vi "Helper - ManualSails.vi"(0 "Full In":bool, 1 "Sheet In":bool, 2 "Sheet Out":bool, 3 "Full Out":bool, 4 "Array":dbl[](array[numeric])) -> (5 "Array 2":dbl[](array[numeric]))   [LabVIEW 2011]
panel:
  # "This is the output array, but it\nnever gets veiwed"
  # "This control gets passed\nan array"
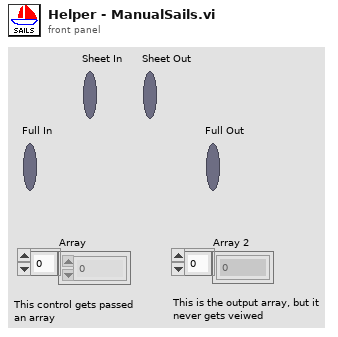
[diagram p1: front panel]
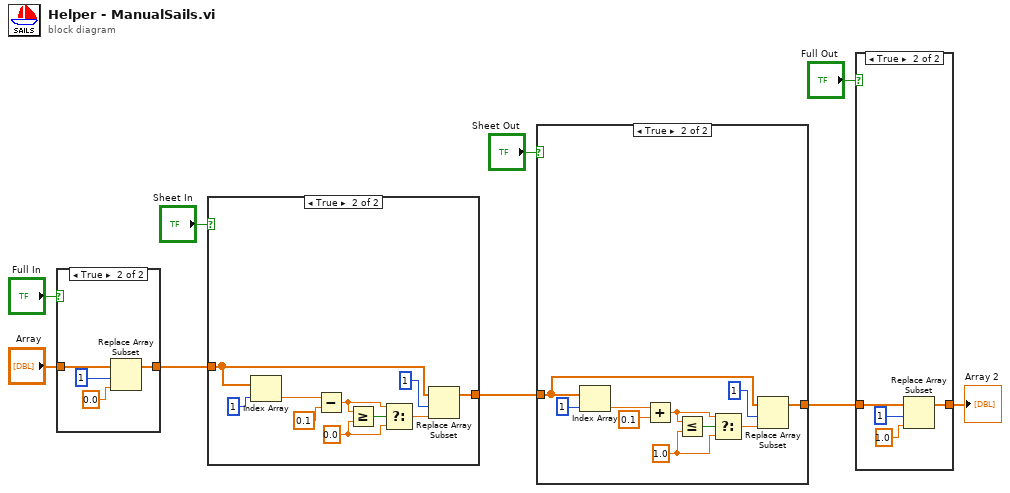
[diagram p0: block diagram]
diagram:
  n1 = case shown="True" "Full In" {
    tunnel: "Array" -> [w10 w14]
    tunnel: [w10 w12] -> w8
    frame False {
    }
    frame True {
      n2 = Replace Array Subset(array=w14, new element=0.0 ("new element/subarray"), index=1) -> (w12:dbl[])
    }
  }
  n3 = case shown="True" "Sheet In" {
    tunnel: w8 -> [w15 w24]
    tunnel: [w15 w25] -> w7
    frame False {
    }
    frame True {
      w20 = 0.0 ("y")
      n4 = Index Array(array=w24, index=1) -> (element=w17:dbl)
      n5 = Subtract(x=w17, y=0.1) -> (x-y=w21:dbl)
      n6 = Greater Or Equal?(x=w21, y=w20) -> (x >= y?=w22:bool)
      n7 = Select(t=w21, s=w22, f=w20) -> (s? t:f=w19:dbl)
      n8 = Replace Array Subset(array=w24, new element=w19, index=1) -> (w25:dbl[])
    }
  }
  n9 = case shown="True" "Sheet Out" {
    tunnel: w7 -> [w26 w35]
    tunnel: [w26 w36] -> w6
    frame False {
    }
    frame True {
      w30 = 1.0 ("y")
      n10 = Index Array(array=w35, index=1) -> (element=w27:dbl)
      n11 = Add(x=w27, y=0.1 ("x")) -> (x+y=w31:dbl)
      n12 = Less Or Equal?(x=w31, y=w30) -> (x <= y?=w32:bool)
      n13 = Select(t=w31, s=w32, f=w30) -> (s? t:f=w29:dbl)
      n14 = Replace Array Subset(array=w35, new element=w29, index=1) -> (w36:dbl[])
    }
  }
  n15 = case shown="True" "Full Out" {
    tunnel: w6 -> [w37 w41]
    tunnel: [w37 w39] -> w5
    frame False {
    }
    frame True {
      n16 = Replace Array Subset(array=w41, new element=1.0 ("new element/subarray"), index=1) -> (w39:dbl[])
    }
  }
  "Array 2" <- w5
